vi "RD Analog In Trigger Source Set.vi"(8 "error in (no error)":errorcluster caption="错误输入（无错误）", 10 "trigsrc":T1(ring), 11 "handle":u64) -> (0 "error out":errorcluster caption="错误输出", 2 "function return":i32, 3 "handle out":u64)   [LabVIEW 2018, in "InstrumentsPlayground.lvlib"]
doc: "CLIFFAPI int CliffAnalogInTriggerSourceSet(FT_HANDLE handle,CLIFFTRIGSRC trigsrc );\ntrigsrc: \nCLIFFTRIGSRCNone = 0;\nCLIFFTRIGSRCDetectorAnalogInCH1 = 1;\nCLIFFTRIGSRCDetectorAnalogInCH2 = 2;\nCLIFFTRIGSRCAnalogOut1 = 3;\nCLIFFTRIGSRCAnalogOut2 = 4;\nCLIFFTRIGSRCDetectorDigitalIn = 5;\nCLIFFTRIGSRCDigitalOut = 6;\nCLIFFTRIGSRCManule = 7;\nCLIFFTRIGSRCExternal1 = 8;\nCLIFFTRIGSRCExternal2 = 9;\nCLIFFTRIGSRCDigitalIn =10;"
uses:
  InstrumentsPlayground.lvlib
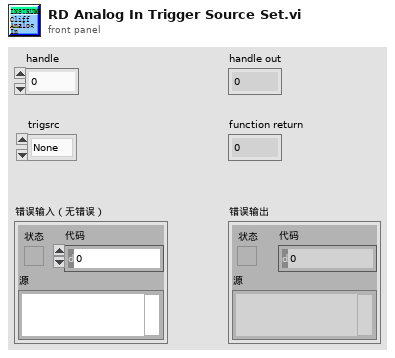
[diagram p1: front panel]
types:
  T1 = enum16{"None", "DetectorAnalogInCH1", "DetectorAnalogInCH2", "AnalogOut1", "AnalogOut2", "DetectorDigitalIn", "DigitalOut", "Manule", "External 1", "External 2", "DigitalIn"}
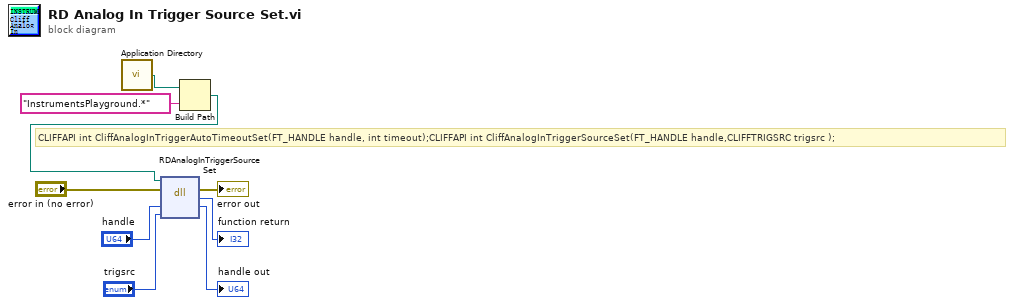
[diagram p0: block diagram]
diagram:
  # "CLIFFAPI int CliffAnalogInTriggerAutoTimeoutSet(FT_HANDLE handle, int timeout);CLIFFAPI int CliffAnalogInTriggerSourceSet(FT_HANDLE handle,CLIFFTRIGSRC trigsrc );"
  n1 = call <vilib>:"Application Directory.vi"() -> ("Application Directory"=w2:path)
  n2 = Build Path(base path=w2, name or relative path="InstrumentsPlayground.*" ("名称或相对路径")) -> (appended path=w1:path)
  n3 = dll-call lib="E:/work/YZCourse_Xtext/Cliff/API/LabVIEW lib/InstrumentsPlayground.*" fn="RDAnalogInTriggerSourceSet"(path in=w1, error in="error in (no error)", "handle"="handle", "trigsrc"="trigsrc") -> (error out=→"error out":errorcluster, "返回类型"=→"function return":i32, "handle"=→"handle out":u64)  [unwired: 2 in, 1 out]
